vi "HFRR ADV v11.vi"() -> ()   [LabVIEW 2025] (continued)
          }
          frame True {
            (unwired) i16 6 ("width (-)")
            (unwired) "TESTED BY : "
            (unwired) "TESTED DATE :"
            (unwired) "SAMPLE ID : "
            (unwired) "SAMPLE DESIGN : "
            w4285 = "\r"
            w4302 = "\r"
            # "add image"
            n3133 = local read "Sample ID"() -> (w4275:string)
            n3134 = local read "Tested by"() -> (w4278:string)
            n3135 = local read "String 34"() -> (w4265:string)
            n3136 = local read "String 45"() -> (w4245:string)
            n3137 = local read "String 35"() -> (w4260:string)
            n3138 = local read "String 37"() -> (w4258:string)
            n3139 = local read "String 32"() -> (w4280:string)
            n3140 = local read "String 36"() -> (w4255:string)
            n3141 = local read "String 31"() -> (w4279:string)
            n3142 = local read "Test Date"() -> (w4276:string)
            n3143 = local read "String 33"() -> (w4281:string)
            n3144 = local read "String 38"() -> (w4251:string)
            n3145 = local read "String 39"() -> (w4248:string)
            n3146 = local write "Print"(FALSE ("Print FF")) -> ()
            n3147 = local read "S 39"() -> (w4263:string)
            n3148 = local read "S 38"() -> (w4270:string)
            n3149 = local read "Temperature before test 2"() -> (w4301:dbl)
            n3150 = local read "Temperature after test 2"() -> (w4291:dbl)
            n3151 = local read "Humidity before test 2"() -> (w4316:dbl)
            n3152 = local read "Humidity after test 2"() -> (w4300:dbl)
            n3153 = local read "MWSD 2"() -> (w4305:dbl)
            n3154 = local read "WS1.4 2"() -> (w4283:dbl)
            n3155 = Concatenate Strings("2)" ("string"), w4265) -> (w4266:string)
            n3156 = Concatenate Strings("3)" ("string"), w4263) -> (w4264:string)
            n3157 = Concatenate Strings("1)" ("string"), w4270) -> (w4269:string)
            n3158 = Concatenate Strings("4)" ("string"), w4260) -> (w4261:string)
            n3159 = Concatenate Strings("5)" ("string"), w4258) -> (w4257:string)
            n3160 = Concatenate Strings("6)" ("string"), w4255) -> (w4254:string)
            n3161 = Concatenate Strings("7)" ("string"), w4251) -> (w4252:string)
            n3162 = Concatenate Strings("8)" ("string"), w4248) -> (w4249:string)
            n3163 = local read "HCF 2"() -> (w4287:dbl)
            n3164 = local read "AVP 2"() -> (w4304:dbl)
            n3165 = local read "s.NO"() -> (w4246:string)
            n3166 = call <vilib>:"New Report.vi"("report type"=enum16{"Standard Report", "HTML"}."Standard Report") -> ("report out"=w4325:refnum<class "NI_report.lvclass">, "error out"=w4324:errorcluster)  [unwired: 13 in]
            n3167 = local read "TITTLE"() -> (w4277:string)
            n3168 = Concatenate Strings(w4302, w4245, w4246, w4302, w4280, w4275, w4302, w4279, w4276, w4302, w4281, w4278, w4302) -> (w4295:string)
            "test by" <- w4295
            n3169 = Number To Fractional String(number=w4301, width (-)=i16 6, precision (6)=i16 2) -> (F-format string=w4290:string)  [unwired: 1 in]
            n3170 = Number To Fractional String(number=w4300, width (-)=i16 6, precision (6)=i16 2) -> (F-format string=w4303:string)  [unwired: 1 in]
            n3171 = Number To Fractional String(number=w4316, width (-)=i16 6, precision (6)=i16 2) -> (F-format string=w4321:string)  [unwired: 1 in]
            n3172 = Number To Fractional String(number=w4305, width (-)=i16 6, precision (6)=i16 2) -> (F-format string=w4307:string)  [unwired: 1 in]
            n3173 = Number To Fractional String(number=w4291, width (-)=i16 6, precision (6)=i16 2) -> (F-format string=w4292:string)  [unwired: 1 in]
            n3174 = Number To Fractional String(number=w4304, width (-)=i16 6, precision (6)=i16 2) -> (F-format string=w4306:string)  [unwired: 1 in]
            n3175 = Number To Fractional String(number=w4287, width (-)=i16 6, precision (6)=i16 2) -> (F-format string=w4286:string)  [unwired: 1 in]
            n3176 = Number To Fractional String(number=w4283, precision (6)=i16 2) -> (F-format string=w4282:string)  [unwired: 2 in]
            n3177 = call-dynamic "Set Report Header Text.vi"("report in"=w4325, "center header text"=w4277, "error in (no error)"=w4324) -> ("report out"=w4296:refnum<class "NI_report.lvclass">, "error out"=w4297:errorcluster)  [unwired: 11 in]
            n3178 = Concatenate Strings(w4285, w4269, w4321, w4285, w4266, w4290, w4285, w4264, w4303, w4285, w4261, w4292, w4285, w4257, w4307, w4285, w4254, w4306, w4285, w4252, w4286, w4285, w4249, w4282) -> (w4273:string)
            "export 2" <- w4273
            n3179 = call-poly <vilib>:"Append Report Text.vi"("report in"=w4296, "text"=w4295, "error in (no error)"=w4297) -> ("report out"=w4299:refnum<class "NI_report.lvclass">, "error out"=w4298:errorcluster)  [unwired: 9 in, 2 out]
            n3180 = local read "test by"() -> (w4272:string)
            n3181 = local read "TITTLE"() -> (w4274:string)
            n3182 = call-poly <vilib>:"Append Report Text.vi"("report in"=w4299, "error in (no error)"=w4298) -> ("report out"=w4320:refnum<class "NI_report.lvclass">, "error out"=w4318:errorcluster)  [unwired: 10 in, 2 out]
            n3183 = Concatenate Strings(w4274, w4273, w4272) -> (→"output":string)
            n3184 = call-poly <vilib>:"Append Report Text.vi"("report in"=w4320, "text"=w4273, "error in (no error)"=w4318) -> ("report out"=w4319:refnum<class "NI_report.lvclass">, "error out"=w4317:errorcluster)  [unwired: 9 in, 2 out]
            n3185 = call-dynamic "Print Report.vi"("report in"=w4319, "printer name (default)"=w4327, "error in (no error)"=w4317) -> ("report out"=w4329:refnum<class "NI_report.lvclass">, "error out"=w4330:errorcluster)  [unwired: 11 in]
            n3186 = call-dynamic "Dispose Report.vi"("report in"=w4329, "error in (no error)"=w4330) -> ()  [unwired: 13 in, 1 out]
          }
        }
        n3187 = case shown="True" "Print 2" {
          frame False {
          }
          frame True {
            n3188 = flat-sequence {
              frame #0 {
                n3189 = local read "s.NO"() -> (→"s.NO 2":string)
                n3190 = Wait (ms)(milliseconds to wait=u32 20) -> ()  [unwired: 1 out]
                n3191 = local read "Sample ID  3"() -> (→"Sample ID  6":string)
                n3192 = local read "Sample ID  4"() -> (→"Sample ID  7":string)
                n3193 = local read "Sample ID"() -> (→"Sample ID  2":string)
                n3194 = local read "Tested by"() -> (→"Tested by 2":string)
                n3195 = local read "Test Date"() -> (→"Test Date 2":string)
                n3196 = local read "Humidity after test 3"() -> (→"Humidity after test 4":dbl)
                n3197 = local read "Ref A Test Date :"() -> (→"TITTLE 4":string)
                n3198 = local read "Temperature before test 3"() -> (w4152:dbl)
                n3199 = local read "Temperature before test 3"() -> (→"Temperature after test 5":dbl)
                n3200 = local read "Temperature after test 3"() -> (→"Temperature after test 4":dbl)
                n3201 = local read "Humidity before test 3"() -> (→"Humidity before test 4":dbl)
                n3202 = local write "Temperature before test 3"(w4152) -> ()
                n3203 = local read "image data"() -> (w4143:T14)
                n3204 = String To Path(string="C:\\LAB-IQ\\im\\Temp_resized.jpg") -> (path=w4144:path)
                "path 2" <- w4144
                n3205 = call <vilib>:"Write JPEG File.vi"("image data"=w4143, "path to JPEG file"=w4144) -> ()  [unwired: 8 in, 2 out]
                "Ref A Test Date :" <- "Ref A Test Date :"
                "Ref B Test Date :" <- "Ref B Test Date :"
                "Ref B Scar Value :" <- "Ref B Scar Value :"
                "Ref A Scar Value :" <- "Ref A Scar Value :"
              }
              frame #1 {
                (unwired) HTML_Report_Image_Alignment."MIDDLE" ("alignment (default)")
                w4180 = u16 0 items=["portrait", "landscape"] ("orientation (portrait)")
                (unwired) HTML_Report_Image_Alignment."ABSMIDDLE" ("alignment (default)")
                (unwired) "TESTED BY : "
                (unwired) "TESTED DATE :"
                (unwired) "SAMPLE ID : "
                (unwired) "SAMPLE DESIGN : "
                w4213 = "\r"
                # "add image"
                n3206 = Wait (ms)(milliseconds to wait=u32 20) -> ()  [unwired: 1 out]
                n3207 = local read "Sample ID  2"() -> (w4206:string)
                n3208 = local read "Wear Scar X"() -> (w4178:dbl)
                "Length ( microns ) 2" <- w4178
                n3209 = local read "Wear Scar Y"() -> (w4177:dbl)
                "Wear Scar Y ( microns ) :" <- w4177
                n3210 = local read "Test Date 2"() -> (w4207:string)
                n3211 = local read "Tested by 2"() -> (w4208:string)
                n3212 = local read "String 46"() -> (w4204:string)
                n3213 = local read "String 48"() -> (w4210:string)
                n3214 = local read "String 47"() -> (w4209:string)
                n3215 = local read "String 49"() -> (w4211:string)
                n3216 = local read "String 10"() -> (w4164:string)
                n3217 = local read "s.NO 2"() -> (w4205:string)
                n3218 = Add(x=w4178, y=w4177) -> (x+y=w4176:dbl)
                n3219 = call <vilib>:"New Report.vi"("report type"=enum16{"Standard Report", "HTML"}."HTML") -> ("report out"=w4184:refnum<class "NI_report.lvclass">, "error out"=w4182:errorcluster)  [unwired: 13 in]
                n3220 = Concatenate Strings(w4213, w4204, w4205, w4213, w4210, w4206, w4213, w4209, w4207, w4213, w4211, w4208, w4213) -> (→"test by 2":string)
                n3221 = Concatenate Strings("C:\\LAB-IQ\\Data\\" ("string"), w4164, ".jpg" ("string")) -> ()  [unwired: 1 out]
                n3222 = Divide(x=w4176, y=2.0) -> (x/y=→"Mean Wear ( microns) :":dbl)
                n3223 = call-dynamic "Set Report Orientation.vi"("report in"=w4184, "orientation (portrait)"=w4180, "error in (no error)"=w4182) -> ("report out"=w4183:refnum<class "NI_report.lvclass">, "error out"=w4181:errorcluster)  [unwired: 11 in]
                n3224 = for {
                  N: 5 -> [_]
                  tunnel: w4183 -> [w4234]
                  tunnel: [w4233] -> w4162
                  tunnel: w4181 -> [w4232]
                  tunnel: [w4231] -> w4161
                  n3225 = call-dynamic "Set Report Tab Width.vi"("report in"=w4234, "error in (no error)"=w4232) -> ("report out"=w4233:refnum<class "NI_report.lvclass">, "error out"=w4231:errorcluster)  [unwired: 12 in]
                }
                n3226 = local read "TITTLE"() -> (w4179:string)
                n3227 = call-dynamic "Set Report Header Text.vi"("report in"=w4162, "center header text"=w4179, "error in (no error)"=w4161) -> ("report out"=w4200:refnum<class "NI_report.lvclass">, "error out"=w4199:errorcluster)  [unwired: 11 in]
                n3228 = for {
                  N: 1 -> [_]
                  tunnel: [w4238] -> w4186
                  tunnel: [w4237] -> w4185
                  tunnel: w4200 -> [w4236]
                  tunnel: w4199 -> [w4235]
                  n3229 = call-dynamic "New Report Line.vi"("report in"=w4236, "error in (no error)"=w4235) -> ("report out"=w4238:refnum<class "NI_report.lvclass">, "error out"=w4237:errorcluster)  [unwired: 12 in]
                }
                n3230 = for {
                  N: 2 -> [_]
                  tunnel: [w4230] -> w4192
                  tunnel: [w4229] -> w4191
                  tunnel: w4186 -> [w4228]
                  tunnel: w4185 -> [w4227]
                  n3231 = call-dynamic "New Report Line.vi"("report in"=w4228, "error in (no error)"=w4227) -> ("report out"=w4230:refnum<class "NI_report.lvclass">, "error out"=w4229:errorcluster)  [unwired: 12 in]
                }
                n3232 = for {
                  N: 25 -> [_]
                  tunnel: w4192 -> [w4226]
                  tunnel: w4191 -> [w4224]
                  tunnel: [w4225] -> w4195
                  tunnel: [w4223] -> w4194
                  n3233 = call-dynamic "Set Report Tab Width.vi"("report in"=w4226, "error in (no error)"=w4224) -> ("report out"=w4225:refnum<class "NI_report.lvclass">, "error out"=w4223:errorcluster)  [unwired: 12 in]
                }
                n3234 = control-ref of="Tab Control 9"() -> (w4190:refnum<vi>)
                n3235 = call-dynamic "Append Control Image to Report.vi"("report in"=w4195, "alignment (default)"=HTML_Report_Image_Alignment."ABSMIDDLE", "ctrl reference"=w4190, "error in (no error)"=w4194) -> ("report out"=w4189:refnum<class "NI_report.lvclass">, "error out"=w4188:errorcluster)  [unwired: 8 in, 2 out]
                n3236 = for {
                  N: 3 -> [_]
                  tunnel: [w4222] -> w4173
                  tunnel: [w4221] -> w4172
                  tunnel: w4189 -> [w4220]
                  tunnel: w4188 -> [w4219]
                  n3237 = call-dynamic "New Report Line.vi"("report in"=w4220, "error in (no error)"=w4219) -> ("report out"=w4222:refnum<class "NI_report.lvclass">, "error out"=w4221:errorcluster)  [unwired: 12 in]
                }
                n3238 = for {
                  N: 100 -> [_]
                  tunnel: w4173 -> [w4218]
                  tunnel: w4172 -> [w4216]
                  tunnel: [w4217] -> w4169
                  tunnel: [w4215] -> w4167
                  n3239 = call-dynamic "Set Report Tab Width.vi"("report in"=w4218, "error in (no error)"=w4216) -> ("report out"=w4217:refnum<class "NI_report.lvclass">, "error out"=w4215:errorcluster)  [unwired: 12 in]
                }
                n3240 = String To Path(string="C:\\LAB-IQ\\im\\Temp_resized.jpg") -> (path=w4159:path)
                n3241 = call-poly <vilib>:"Append Image to Report.vi"("report in"=w4169, "path or URL of image"=w4159, "error in (no error)"=w4167) -> ("report out"=w4168:refnum<class "NI_report.lvclass">, "error out"=w4166:errorcluster)  [unwired: 9 in, 2 out]
                n3242 = call-poly <vilib>:"Open HTML Report in Browser.vi"("report in"=w4168, "error in (no error)"=w4166) -> ("report out"=w4203:refnum<class "NI_report.lvclass">, "error out"=w4202:errorcluster)  [unwired: 11 in, 1 out]
                n3243 = call-dynamic "Dispose Report.vi"("report in"=w4203, "error in (no error)"=w4202) -> ()  [unwired: 13 in, 1 out]
              }
              frame #2 {
              }
              frame #3 {
                n3244 = disable-structure shown="Disabled" {
                  frame Disabled {
                    n3245 = local read "String 10"() -> (w4243:string)
                    n3246 = Concatenate Strings("C:\\LAB-IQ-NXT\\Data\\" ("string"), w4243, ".jpg" ("string")) -> (w4241:string)
                    n3247 = String To Path(string=w4241) -> (path=w4240:path)
                    n3248 = Delete(path (use dialog)=w4240) -> ()  [unwired: 4 in, 3 out]
                  }
                  frame Enabled {
                  }
                }
                n3249 = local write "Print 2"(FALSE ("Print")) -> ()
              }
            }
          }
        }
      }
    }
    n3250 = property on="SetTemp" class="DigNum (strict)"("Disabled"=w2127) -> ()  [unwired: 2 in, 2 out]
    n3251 = Multiply(x=w2116, y=w2118) -> (x*y=w2117:dbl)
    n3252 = local read "MWSD"() -> (w2115:dbl)
    n3253 = Add(x=w2117, y=w2115) -> (x+y=→"WS1.4":dbl)
    n3254 = Wait (ms)(milliseconds to wait=u32 50) -> ()  [unwired: 1 out]
    n3255 = Wait (ms)(milliseconds to wait=u32 50) -> ()  [unwired: 1 out]
    n3256 = local read "Quit"() -> (w2114:bool)
  }
  n3257 = VISA Close(VISA resource name=w53, error in (no error)=w52) -> (error out=w50:errorcluster)
  n3258 = VISA Close(VISA resource name=w34, error in (no error)=w33) -> ()  [unwired: 1 out]
  n3259 = call <vilib>:"Clear Errors.vi"("error in (no error)"=w50) -> ()  [unwired: 5 in, 2 out]
  n3260 = Or(x=w40, y=w39) -> (x .or. y?=w41:bool)
  n3261 = while {
    tunnel: [w4391] -> w46
    shift-right: [w4429] -> _
    shift-left: "" -> [w4417]
    tunnel: [w4405] -> _
    i -> [w4405]
    stop <- w4391 stop-if-true
    w4431 = ";" ("string")
    n3262 = local read "start en"() -> (w4450:bool)
    n3263 = And(x="st enable", y=w4450) -> (x .and. y?=w4451:bool)
    n3264 = local read "Elapsed time"() -> (w4413:dbl)
    n3265 = local read "ACQUIRE 3"() -> (w4394:bool)
    n3266 = case shown="True" w4451 {
      tunnel: "st enable" -> [w4515 w4516]
      tunnel: [w4515 w4516] -> w4395
      frame False {
      }
      frame True {
        n3267 = local write "start en"(FALSE ("start en")) -> ()
      }
    }
    n3268 = Wait (ms)(milliseconds to wait=u32 80) -> ()  [unwired: 1 out]
    n3269 = local read "Stroke"() -> (w4404:dbl)
    n3270 = Greater?(x=w4413, y=0.1) -> (0:w4411:bool)
    n3271 = Or(x=w4395, y=w4394) -> (x .or. y?=w4396:bool)
    n3272 = case shown="True" "ACQUIRE 2" {
      frame False {
      }
      frame True {
        n3273 = call "Elapsed Time13"() -> ("Time has Elapsed"=w4458:bool)  [unwired: 12 in, 7 out]
        n3274 = case shown="True" w4458 {
          frame False {
          }
          frame True {
            n3275 = local write "ACQUIRE 2"(FALSE ("ACQUIRE 2")) -> ()
            n3276 = local write "ACQUIRE 3"(FALSE ("ACQUIRE 2")) -> ()
          }
        }
        n3277 = local write "ACQUIRE 3"(TRUE ("ACQUIRE 2")) -> ()
      }
    }
    n3278 = case shown="True" w4396 {
      tunnel: w4404 -> [_ w4538]
      tunnel: [w4518 _] -> w4448
      tunnel: w4411 -> [_ _]
      tunnel: w4394 -> [_ w4525]
      frame False {
        w4518 = TRUE ("PID Rst")
        n3279 = local read "stop cmd"() -> (w4519:bool)
        n3280 = case shown="True" w4519 {
          frame False {
          }
          frame True {
            n3281 = local write "stop cmd"(FALSE ("stop cmd")) -> ()
          }
        }
        n3282 = local write "PID Rst"(TRUE ("PID Rst")) -> ()
        "start en" <- w4518
      }
      frame True {
        w4545 = cluster{"output high":dbl, "output low":dbl} {"output high"=600.0, "output low"=-600.0} ("output range")
        n3283 = local read "STROKE GAIN :"() -> (w4530:dbl)
        n3284 = call "Elapsed Time6"("Reset"="PID Rst", "Auto Reset"=FALSE) -> ("Time has Elapsed"=w4539:bool)  [unwired: 10 in, 7 out]
        n3285 = Multiply(x="Set Strk", y=w4530) -> (x*y=w4523:dbl)
        n3286 = case shown="False" w4539 {
          tunnel: [w4550 w4551] -> w4542
          tunnel: "Set Strk" -> [w4550 _]
          tunnel: w4538 -> [_ w4551]
          frame False {
          }
          frame True {
          }
        }
        n3287 = Multiply(x=w4523, y=1.0) -> (x*y=w4522:dbl)
        n3288 = Select(t=T9 {"Proportional Gain (Kc)"=0.0, "Integral Time (Ti, min)"=0.02, "Derivative Time (Td, min)"=0.0} ("Stroke PID Gains"), s=w4525, f="Stroke PID Gains") -> (s? t:f=w4526:T9)
        n3289 = Not(x=w4539) -> (.not. x?=w4537:bool)
        n3290 = call-poly <vilib>:"PID.vi"("reinitialize? (F)"=w4537, "output range"=w4545, "PID gains"=w4526, "process variable"=w4542, "setpoint"="Set Strk") -> ("output"=w4536:dbl)  [unwired: 5 in, 1 out]
        "Stroke PID OUT" <- w4536
        n3291 = Select(t=w4536, s=w4539, f=0.0) -> (s? t:f=w4540:dbl)
        n3292 = flat-sequence {
          tunnel: w4540 -> [_]
          frame #0 {
            n3293 = local write "PID Rst"(FALSE ("PID Rst")) -> ()
          }
        }
        n3294 = Add(x=w4522, y=w4540) -> (x+y=w4535:dbl)
        n3295 = Unbundle(w4545) -> ("output high"=w4544:dbl, "output low"=w4543:dbl)
        n3296 = To Word Integer(number=w4535) -> (16bit integer=w4532:i16)
        n3297 = property on="Stroke PID OUT" class="Slide (strict)"("Scale.Range:Minimum"=w4543, "Scale.Range:Maximum"=w4544) -> ()  [unwired: 2 in, 2 out]
        n3298 = In Range and Coerce(upper limit=4095.0 ("f"), x=w4532, lower limit=100.0 ("f")) -> (coerced(x)=w4529:dbl)  [unwired: 1 out]
        "PID Out" <- w4529
        n3299 = Number To Decimal String(number=w4529) -> (decimal integer string=→"st gain":string)  [unwired: 1 in]
        "stop cmd" <- TRUE ("Auto Reset")
      }
    }
    n3300 = flat-sequence {
      frame #0 {
        n3301 = local read "CH-POWER +"() -> (w4462:u16)
        n3302 = local read "CH-POWER -"() -> (w4463:u16)
        n3303 = case shown="1" w4463 {
          tunnel: "PWR" -> [w4464 w4465 w4466 w4467 w4468 w4469 w4470 w4471]
          frame 0, Default {
            n3304 = local write "Do 0"(w4464) -> ()
          }
          frame 1 {
            n3305 = local write "Do 1"(w4465) -> ()
          }
          frame 2 {
            n3306 = local write "Do 2"(w4466) -> ()
          }
          frame 3 {
            n3307 = local write "Do 3"(w4467) -> ()
          }
          frame 4 {
            n3308 = local write "Do 4"(w4468) -> ()
          }
          frame 5 {
            n3309 = local write "Do 5"(w4469) -> ()
          }
          frame 6 {
            n3310 = local write "Do 6"(w4470) -> ()
          }
          frame 7 {
            n3311 = local write "Do 7"(w4471) -> ()
          }
        }
        n3312 = case shown="1" w4462 {
          tunnel: "PWR" -> [w4472 w4473 w4474 w4475 w4476 w4477 w4478 w4479]
          frame 0, Default {
            n3313 = local write "Do 0"(w4472) -> ()
          }
          frame 1 {
            n3314 = local write "Do 1"(w4473) -> ()
          }
          frame 2 {
            n3315 = local write "Do 2"(w4474) -> ()
          }
          frame 3 {
            n3316 = local write "Do 3"(w4475) -> ()
          }
          frame 4 {
            n3317 = local write "Do 4"(w4476) -> ()
          }
          frame 5 {
            n3318 = local write "Do 5"(w4477) -> ()
          }
          frame 6 {
            n3319 = local write "Do 6"(w4478) -> ()
          }
          frame 7 {
            n3320 = local write "Do 7"(w4479) -> ()
          }
        }
      }
    }
    n3321 = local read "RUN"() -> (w4402:bool)
    n3322 = Or(x=w4402, y="ACQUIRE 3") -> (x .or. y?=w4401:bool)
    n3323 = local read "Set Hz"() -> (w4419:dbl)
    n3324 = Select(t=w4419, s=w4401, f=0.0) -> (s? t:f=w4418:dbl)
    n3325 = local read "st gain"() -> (w4422:string)
    n3326 = local read "DO"() -> (w4423:string)
    n3327 = case shown="True" "Boolean 10" {
      frame False {
      }
      frame True {
        n3328 = local write "Tab Control 8"(enum32{"setup", "calibrate"}."calibrate" ("Tab Control 8")) -> ()
        n3329 = local write "Boolean 10"(FALSE ("Boolean 10")) -> ()
      }
    }
    n3330 = Number To Decimal String(number=w4418) -> (decimal integer string=w4421:string)  [unwired: 1 in]
    n3331 = case shown="True" "Boolean 11" {
      frame False {
      }
      frame True {
        n3332 = local write "Tab Control 8"(enum32{"setup", "calibrate"}."setup" ("Tab Control 8")) -> ()
        n3333 = local write "Boolean 11"(FALSE ("Boolean 11")) -> ()
      }
    }
    n3334 = String Length(string=w4422) -> (length=w4437:i32)
    n3335 = String Length(string=w4423) -> (length=w4425:i32)
    n3336 = String Length(string=w4421) -> (length=w4438:i32)
    n3337 = Subtract(x=4.0, y=w4437) -> (x-y=w4434:dbl)
    n3338 = Subtract(x=3.0, y=w4425) -> (x-y=w4428:dbl)
    n3339 = flat-sequence {
      tunnel: w4448 -> [_]
      frame #0 {
        n3340 = Build Array("Do 0", "Do 1", "Do 2", "Do 3", "Do 4", "Do 5", "Do 6", "Do 7") -> (w4506:bool[])
        n3341 = Boolean Array To Number(Boolean array=w4506) -> (number=w4504:u32)
        n3342 = Add(x=w4504, y=u32 0) -> (x+y=w4502:u32)
        n3343 = Number To Decimal String(number=w4502) -> (decimal integer string=→"DO":string)  [unwired: 1 in]
      }
    }
    n3344 = Subtract(x=3.0, y=w4438) -> (x-y=w4439:dbl)
    n3345 = Replace Substring(3:w4434, 4:w4422, 5:"0000" ("string")) -> (1:w4432:string)  [unwired: 1 in, 1 out]
    n3346 = Replace Substring(3:w4428, 4:w4423, 5:"000" ("string")) -> (1:w4424:string)  [unwired: 1 in, 1 out]
    n3347 = Replace Substring(3:w4439, 4:w4421, 5:"000" ("string")) -> (1:w4433:string)  [unwired: 1 in, 1 out]
    n3348 = Concatenate Strings("*" ("string"), w4433, w4431, w4432, w4431, w4424, "$" ("string")) -> (w4429:string)
    "Stroke_send_Val" <- w4429
    n3349 = local read "RUN"() -> (w4399:bool)
    n3350 = local read "ACQUIRE 3"() -> (w4398:bool)
    n3351 = local read "send"() -> (w4415:bool)
    n3352 = Not Equal?(x=w4417, y=w4429) -> (x != y?=w4430:bool)
    n3353 = Or(x=w4399, y=w4398) -> (x .or. y?=w4397:bool)
    n3354 = And(x=w4415, y=w4397) -> (x .and. y?=w4414:bool)
    n3355 = Or(x=w4430, y=w4414) -> (x .or. y?=w4408:bool)
    n3356 = case shown="False" w4397 {
      frame False {
        "send" <- TRUE ("send")
      }
      frame True {
      }
    }
    n3357 = call "Elapsed Time4"("Time Target (s)"=0.5) -> ("Time has Elapsed"=w4406:bool)  [unwired: 11 in, 7 out]
    n3358 = local read "Din"() -> (w4447:u8[])
    n3359 = Or(x=w4406, y=w4408) -> (x .or. y?=w4407:bool)
    n3360 = local read "Quit"() -> (w4391:bool)
    n3361 = Index Array(array=w4447, index=0) -> (element=w4445:u8)
    n3362 = case shown="True" w4407 {
      tunnel: w4429 -> [_ w4483]
      frame False {
      }
      frame True {
        n3363 = local read "Due Com"() -> (w4484:string[])
        n3364 = Build Array (concatenate)(w4484, w4483) -> (→"Due Com":string[])
        n3365 = local write "send"(FALSE ("send")) -> ()
      }
    }
    n3366 = Number To Boolean Array(number=w4445) -> (Boolean array=w4444:bool[])
    n3367 = Array Size(array=w4444) -> (size(s)=w4443:i32)
    n3368 = Greater Than 0?(x=w4443) -> (x > 0?=w4442:bool)
    n3369 = case shown="True" w4442 {
      tunnel: w4444 -> [_ w4498]
      frame False {
      }
      frame True {
        n3370 = Index Array(array=w4498, index #1=0 ("index"), index #2=1 ("index"), index #3=2 ("index"), index #4=3 ("index"), index #5=4 ("index"), index #6=5 ("index"), index #7=6 ("index"), index #8=7 ("index")) -> (element #1=→"DI 0":bool, element #2=→"DI 1":bool, element #3=→"DI 2":bool, element #4=→"DI 3":bool, element #5=→"DI 4":bool, element #6=→"DI 5":bool, element #7=→"DI 6":bool, element #8=→"DI 7":bool)
      }
    }
  }
  n3371 = Or(x=w36, y=w41) -> (x .or. y?=w48:bool)
  n3372 = control-ref of="new picture"() -> ()  [unwired: 1 out]
  n3373 = Or(x=w55, y=w48) -> (x .or. y?=w45:bool)
  n3374 = Or(x=w45, y=w46) -> (x .or. y?=w37:bool)
  n3375 = while {
    tunnel: [w4553] -> w59
    tunnel: [w4554] -> _
    i -> [w4554]
    stop <- w4553 stop-if-true
    n3376 = local read "PID-out"() -> (w4555:dbl)
    "Horizontal Slider Control" <- w4555
    n3377 = Greater Or Equal?(x=w4555, y=2.0) -> (x >= y?=w4556:bool)
    n3378 = flat-sequence {
      tunnel: w4556 -> [w4564]
      tunnel: w4555 -> [w4567]
      tunnel: [w4565] -> w4562
      tunnel: [w4563] -> w4561
      tunnel: [w4583] -> w4560
      tunnel: w4562 -> [w4583]
      tunnel: w4561 -> [w4580]
      tunnel: [w4580] -> w4559
      tunnel: w4560 -> [w4585]
      tunnel: [w4584] -> w4558
      tunnel: w4559 -> [w4584]
      tunnel: w4558 -> [w4599]
      frame #0 {
        n3379 = case shown="True" w4564 {
          selector: w4564 -> [w4569 _]
          frame False {
            n3380 = local write "HEATER"(w4569) -> ()
          }
          frame True {
            w4571 = TRUE ("data")
            n3381 = local read "CH-HEATER"() -> (w4570:u16)
            n3382 = case shown="2" w4570 {
              tunnel: w4571 -> [w4572 w4573 w4574 w4575 w4576 w4577 w4578 w4579]
              frame 0, Default {
                n3383 = local write "Do 0"(w4572) -> ()
              }
              frame 1 {
                n3384 = local write "Do 1"(w4573) -> ()
              }
              frame 2 {
                n3385 = local write "Do 2"(w4574) -> ()
              }
              frame 3 {
                n3386 = local write "Do 3"(w4575) -> ()
              }
              frame 4 {
                n3387 = local write "Do 4"(w4576) -> ()
              }
              frame 5 {
                n3388 = local write "Do 5"(w4577) -> ()
              }
              frame 6 {
                n3389 = local write "Do 6"(w4578) -> ()
              }
              frame 7 {
                n3390 = local write "Do 7"(w4579) -> ()
              }
            }
            "HEATER" <- w4571
          }
        }
        n3391 = Select(t=w4567, s=w4564, f=0.0) -> (s? t:f=w4563:dbl)
        n3392 = Greater Or Equal?(x=w4567, y=97.0) -> (x >= y?=w4565:bool)
      }
      frame #1 {
        n3393 = Multiply(x=w4580, y=5.0) -> (x*y=w4582:dbl)
        n3394 = Wait (ms)(milliseconds to wait=w4582) -> ()  [unwired: 1 out]
      }
      frame #2 {
        n3395 = case shown="False" w4585 {
          frame False {
            w4586 = FALSE ("data")
            n3396 = local read "CH-HEATER"() -> (w4587:u16)
            n3397 = case shown="4" w4587 {
              tunnel: w4586 -> [w4588 w4589 w4590 w4591 w4592 w4593 w4594 w4595]
              frame 0, Default {
                n3398 = local write "Do 0"(w4588) -> ()
              }
              frame 1 {
                n3399 = local write "Do 1"(w4589) -> ()
              }
              frame 2 {
                n3400 = local write "Do 2"(w4590) -> ()
              }
              frame 3 {
                n3401 = local write "Do 3"(w4591) -> ()
              }
              frame 4 {
                n3402 = local write "Do 4"(w4592) -> ()
              }
              frame 5 {
                n3403 = local write "Do 5"(w4593) -> ()
              }
              frame 6 {
                n3404 = local write "Do 6"(w4594) -> ()
              }
              frame 7 {
                n3405 = local write "Do 7"(w4595) -> ()
              }
            }
            n3406 = local write "HEATER"(w4586) -> ()
          }
          frame True {
          }
        }
      }
      frame #3 {
        n3407 = Subtract(x=100, y=w4599) -> (x-y=w4598:dbl)
        n3408 = Multiply(x=w4598, y=5.0) -> (x*y=w4596:dbl)
        n3409 = Wait (ms)(milliseconds to wait=w4596) -> ()  [unwired: 1 out]
      }
    }
    n3410 = local read "Quit"() -> (w4553:bool)
  }
  n3411 = Or(x=w59, y=w37) -> (x .or. y?=w58:bool)
  n3412 = while {
    tunnel: [w4601] -> w54
    i -> [w4608]
    stop <- w4601 stop-if-true
    n3413 = local read "Quit"() -> (w4601:bool)
    n3414 = Equal To 0?(x=w4608) -> (x = 0?=w4606:bool)
    n3415 = call "Elapsed Time3"("Time Target (s)"=45.0, "Auto Reset"=TRUE) -> ("Time has Elapsed"=w4605:bool)  [unwired: 10 in, 7 out]
    n3416 = Wait (ms)(milliseconds to wait=u32 50) -> ()  [unwired: 1 out]
    n3417 = Or(x=w4605, y=w4606) -> (x .or. y?=w4607:bool)
    n3418 = case shown="True" w4607 {
      frame False {
      }
      frame True {
        n3419 = call <vilib>:"System Exec.vi"("run minimized? (F)"=TRUE, "error in (no error)"="error in (no error)", "command line"="powercfg.exe -change -monitor-timeout-ac 0") -> ("error out"=w4619:errorcluster)  [unwired: 5 in, 3 out]
        n3420 = call <vilib>:"System Exec.vi"("run minimized? (F)"=TRUE, "error in (no error)"=w4619, "command line"="powercfg.exe -change -disk-timeout-ac 0") -> ("error out"=w4618:errorcluster)  [unwired: 5 in, 3 out]
        n3421 = call <vilib>:"System Exec.vi"("run minimized? (F)"=TRUE, "error in (no error)"=w4618, "command line"="powercfg.exe -change -standby-timeout-ac 0") -> ("error out"=w4617:errorcluster)  [unwired: 5 in, 3 out]
        n3422 = call <vilib>:"System Exec.vi"("run minimized? (F)"=TRUE, "error in (no error)"=w4617, "command line"="powercfg.exe -change -hibernate-timeout-ac 0") -> ("error out"=w4616:errorcluster)  [unwired: 5 in, 3 out]
        n3423 = call <vilib>:"Simple Error Handler.vi"("error in (no error)"=w4616) -> ("error out"=w4622:errorcluster)  [unwired: 4 in, 4 out]
        n3424 = call <vilib>:"Clear Errors.vi"("error in (no error)"=w4622) -> ("error out"=→"error out":errorcluster)  [unwired: 5 in, 1 out]
      }
    }
  }
  n3425 = Compound Arithmetic op=OR(w57, w58, w54) -> (w56:bool)
  n3426 = flat-sequence {
    tunnel: w56 -> [_]
    tunnel: [w4624] -> w14
    tunnel: w14 -> [_]
    frame #0 {
      n3427 = call "CLOSE CONNECTION.vi"() -> ("error out"=w4624:errorcluster)  [unwired: 11 in]
    }
    frame #1 {
      n3428 = Quit LabVIEW(quit? (T)=TRUE) -> ()
      n3429 = local write "Quit"(FALSE ("EXIT")) -> ()
    }
  }
  n3430 = property on="Heater Button" class="Bool (strict)"("Visible"=TRUE) -> ()  [unwired: 2 in, 2 out]
  n3431 = disable-structure shown="Disabled" {
    disable-tunnel: _ -> [w4630 _]
    disable-tunnel: _ -> [w4627 _]
    disable-tunnel: _ -> [w4628 _]
    frame Disabled {
      n3432 = disable-structure shown="Disabled" {
        disable-tunnel: [w4637 _] -> w4629
        frame Disabled {
          n3433 = while {
            shift-right: [w4679] -> w4635
            shift-left: errorcluster {"status"=TRUE, "code"=0, "source"="Init"} ("error out") -> [w4644]
            shift-right: [w4678] -> w4634
            shift-left: _ -> [w4645]
            shift-right: [w4677] -> _
            shift-left: "" -> [w4676]
            tunnel: [w4638] -> w4637
            shift-right: ["Set Rh"] -> _
            shift-left: 0.0 ("Set Rh") -> [w4670]
            tunnel: [w4647] -> _
            i -> [w4647]
            stop <- w4638 stop-if-true
            n3434 = flat-sequence {
              tunnel: w4644 -> [w4682]
              tunnel: [w4682] -> w4643
              frame #0 {
                n3435 = Wait (ms)(milliseconds to wait=u32 200) -> ()  [unwired: 1 out]
              }
            }
            n3436 = local read "Com Port 3"() -> (w4646:refnum<visa-resource-name>)
            n3437 = local read "Humidity Str Rec"() -> (w4648:string)
            n3438 = Not Equal?(x="Set Rh", y=w4670) -> (x != y?=w4675:bool)
            n3439 = Number To Decimal String(number="Set Rh") -> (decimal integer string=w4673:string)  [unwired: 1 in]
            n3440 = Not Equal?(x=w4646, y=w4645) -> (x != y?=w4641:bool)
            n3441 = Concatenate Strings("#setPoint00" ("string"), w4673) -> (w4674:string)
            n3442 = case shown="False" w4675 {
              tunnel: w4674 -> [_ w4694]
              frame False {
                n3443 = local read "Humidity"() -> (w4691:bool)
                n3444 = case shown="True" w4691 {
                  frame False {
                    n3445 = local write "Humidity Str Send"("stop" ("Humidity Str Send")) -> ()
                  }
                  frame True {
                    n3446 = local write "Humidity Str Send"("start" ("Humidity Str Send")) -> ()
                  }
                }
              }
              frame True {
                n3447 = local write "Humidity Str Send"(w4694) -> ()
              }
            }
            n3448 = Or(x=w4641, y="Re-Initialise") -> (x .or. y?=w4640:bool)
            n3449 = String Subset(string=w4648, offset (0)=7) -> (substring=w4663:string)  [unwired: 1 in]
            n3450 = Match Pattern(string=w4648, regular expression="?") -> (offset past match=w4666:i32)  [unwired: 1 in, 3 out]
            n3451 = Match Pattern(string=w4648, regular expression="v") -> (offset past match=w4669:i32)  [unwired: 1 in, 3 out]
            n3452 = case shown="True" w4640 {
              tunnel: w4643 -> [w4680 _]
              tunnel: [w4680 errorcluster {"status"=TRUE, "code"=0, "source"="Init"} ("error out")] -> w4642
              frame False {
              }
              frame True {
              }
            }
            n3453 = Equal?(x=w4666, y=-1) -> (x = y?=w4650:bool)
            n3454 = Match Pattern(string=w4663, regular expression="g") -> (after substring=w4664:string, offset past match=w4655:i32)  [unwired: 1 in, 2 out]
            n3455 = Match Pattern(string=w4663, regular expression="y") -> (after substring=w4662:string, offset past match=w4656:i32)  [unwired: 1 in, 2 out]
            n3456 = Greater?(x=w4656, y=w4655) -> (0:w4661:bool)
            n3457 = Greater Or Equal To 0?(x=w4656) -> (x >= 0?=w4653:bool)
            n3458 = Greater Or Equal To 0?(x=w4655) -> (x >= 0?=w4654:bool)
            n3459 = Or(x=w4653, y=w4654) -> (x .or. y?=w4652:bool)
            n3460 = Greater Or Equal To 0?(x=w4669) -> (x >= 0?=w4651:bool)
            n3461 = Select(t=w4662, s=w4661, f=w4664) -> (s? t:f=w4657:string)
            n3462 = case shown="Error" w4642 {
              selector: w4642 -> [w4707 w4753]
              tunnel: [w4705 w4746] -> w4679
              tunnel: w4645 -> [w4708 w4752]
              tunnel: [w4706 w4755] -> w4678
              tunnel: w4676 -> [w4695 w4754]
              tunnel: [w4702 w4754] -> w4677
              frame No Error {
                n3463 = call "Elapsed Time7"() -> ("Time has Elapsed"=w4701:bool)  [unwired: 12 in, 7 out]
                n3464 = Not Equal?(x="Humidity Str Send", y=w4695) -> (x != y?=w4697:bool)
                n3465 = Or(x=w4697, y=w4701) -> (x .or. y?=w4700:bool)
                n3466 = Select(t="Humidity Str Send", s=w4697, f="vals" ("regular expression")) -> (s? t:f=w4696:string)
                n3467 = Or(x=w4700, y="Send") -> (x .or. y?=w4704:bool)
                n3468 = case shown="True" w4704 {
                  tunnel: [w4711 w4716] -> w4705
                  tunnel: w4708 -> [w4710 w4724]
                  tunnel: w4707 -> [w4711 w4723]
                  tunnel: [w4710 w4717] -> w4706
                  tunnel: w4696 -> [_ w4722]
                  tunnel: [w4709 w4713] -> w4702
                  tunnel: "Humidity Str Send" -> [_ w4714]
                  tunnel: w4697 -> [_ w4715]
                  tunnel: w4695 -> [w4709 w4712]
                  frame False {
                  }
                  frame True {
                    n3469 = flat-sequence {
                      tunnel: w4724 -> [w4732]
                      tunnel: w4723 -> [w4731]
                      tunnel: w4722 -> [w4728]
                      tunnel: [w4730] -> w4721
                      tunnel: [w4729] -> w4720
                      tunnel: w4721 -> [w4735]
                      tunnel: w4720 -> [w4734]
                      tunnel: [w4735] -> w4719
                      tunnel: [w4734] -> w4718
                      tunnel: w4719 -> [w4742]
                      tunnel: w4718 -> [w4741]
                      tunnel: [w4740] -> w4717
                      tunnel: [w4739] -> w4716
                      frame #0 {
                        n3470 = local write "Ser Led"(TRUE ("Boolean 4")) -> ()
                        n3471 = Concatenate Strings(w4728, "\r") -> (w4727:string)
                        n3472 = VISA Write(VISA resource name=w4732, write buffer=w4727, error in (no error)=w4731) -> (VISA resource name out=w4730:refnum<visa-resource-name>, error out=w4729:errorcluster)  [unwired: 1 out]
                      }
                      frame #1 {
                        n3473 = Wait (ms)(milliseconds to wait="wait") -> ()  [unwired: 1 out]
                      }
                      frame #2 {
                        w4737 = FALSE ("Send")
                        n3474 = property class="Instr"(reference=w4742, error in=w4741) -> (reference out=w4743:refnum<visa-resource-name>, error out=w4744:errorcluster, "Serial Settings:Number of Bytes at Serial Port"=w4736:u32)
                        "Humidity 2" <- w4736
                        n3475 = local write "Send"(w4737) -> ()
                        n3476 = local write "Ser Led"(w4737) -> ()
                        n3477 = VISA Read(VISA resource name=w4743, byte count=w4736, error in (no error)=w4744) -> (VISA resource name out=w4740:refnum<visa-resource-name>, read buffer=→"Humidity Str Rec":string, error out=w4739:errorcluster)  [unwired: 1 out]
                      }
                    }
                    n3478 = Select(t=w4714, s=w4715, f=w4712) -> (s? t:f=w4713:string)
                  }
                }
              }
              frame Error {
                w4760 = u16 0 items=["None"=0, "XON/XOFF"=1, "RTS/CTS"=2, "DTR/DSR"=4] ("flow control")
                w4756 = u16 0 items=["None", "Odd", "Even", "Mark", "Space"] ("parity")
                w4759 = u16 10 items=["1.0"=10, "1.5"=15, "2.0"=20] ("stop bits")
                n3479 = VISA Close(VISA resource name=w4752, error in (no error)=w4753) -> (error out=w4751:errorcluster)
                n3480 = local write "humid"("" ("humid")) -> ()
                n3481 = local write "Humidity Str Rec"("" ("Humidity Str Rec")) -> ()
                n3482 = call <vilib>:"Clear Errors.vi"("error in (no error)"=w4751) -> ("error out"=w4750:errorcluster)  [unwired: 5 in, 1 out]
                n3483 = local read "Com Port 3"() -> (w4749:refnum<visa-resource-name>)
                n3484 = call-poly "VISA Configure Serial Port"("VISA resource name"=w4749, "timeout (10sec)"=u32 1000, "termination char\n(0xA = '\\n' = LF)"=u8 10 ("termination char\n(0xA = '\\n' = LF)"), "Enable Termination\nChar (T)"=FALSE ("Enable Termination Char (T)"), "baud rate (9600)"="Humidity BaudRate", "data bits (8)"=u16 8 ("data bits"), "parity (0:none)"=w4756, "error in (no error)"=w4750, "stop bits (10: 1 bit)"=w4759, "flow control (0:none)"=w4760) -> ("VISA resource name out"=w4755:refnum<visa-resource-name>, "error out"=w4746:errorcluster)  [unwired: 4 in]
              }
            }
            n3485 = Compound Arithmetic op=AND(w4651, w4650, w4652) -> (w4649:bool)
            n3486 = case shown="True" w4649 {
              tunnel: w4648 -> [_ _]
              tunnel: w4657 -> [_ w4687]
              frame False {
              }
              frame True {
                w4685 = " " ("regular expression")
                n3487 = Match Pattern(string=w4687, regular expression=" ") -> (after substring=w4689:string)  [unwired: 1 in, 3 out]
                n3488 = Match Pattern(string=w4689, regular expression=w4685) -> (before substring=→"humid":string, after substring=w4686:string)  [unwired: 1 in, 2 out]
                n3489 = Match Pattern(string=w4686, regular expression=w4685) -> (before substring=→"temp_@Rh sensor":string)  [unwired: 1 in, 3 out]
              }
            }
            n3490 = local read "Quit"() -> (w4638:bool)
          }
          n3491 = VISA Close(VISA resource name=w4634, error in (no error)=w4635) -> (error out=w4631:errorcluster)
          n3492 = call <vilib>:"Clear Errors.vi"("error in (no error)"=w4631) -> ()  [unwired: 5 in, 2 out]
        }
        frame Enabled {
        }
      }
    }
    frame Enabled {
    }
  }
  n3493 = while {
    tunnel: [w4768] -> _
    i -> [w4768]
    stop <- w4763 stop-if-true
    # "Langauage selection"
    n3494 = property on="FF Calibration g" class="WFGraph (strict)"("Plot Area:Colors:FG Color"=u32 0) -> ()  [unwired: 2 in, 2 out]
    n3495 = Equal?(x="Lan flag", y=22.0) -> ()  [unwired: 1 out]
    n3496 = disable-structure shown="Disabled" {
      frame Disabled {
        n3497 = stacked-sequence {
          frame #0 {
            n3498 = case shown="\"Russian\"" "Language Selection" {
              tunnel: [0 1] -> w4770
              frame "English", Default {
              }
              frame "Russian" {
              }
            }
            n3499 = for {
              N: 130 -> [_]
              tunnel: "Table" -> [w4779]
              tunnel: w4770 -> [w4778]
              i -> [w4777]
              n3500 = Index Array(array=w4779, index (row)=w4777, index (col)=w4778) -> (element=w4776:string)
              n3501 = case shown="4" w4777 {
                tunnel: w4776 -> [w4780 w4781 _ w4782 w4783 w4784 w4785 w4786 w4787 w4788 w4789 w4790 w4791 w4792 w4793 w4794 w4795 w4796 w4797 w4798 w4799 w4800 w4801 w4802 w4803 w4804 w4805 w4806 w4807 _ _ w4808 w4809 w4810 w4811 w4812 w4813 w4822 w4829 w4836 w4843 w4847 w4850 w4853 w4855 w4857 w4858 w4859 w4860 w4861 w4862 w4863 w4864 w4865 w4866 w4867 w4868 w4869 w4870 w4871 w4872 w4873 w4874 w4875 w4876 w4877 w4878 w4879 w4880 w4881 w4882 w4883 w4884 w4885 w4886 w4887 w4888 w4889 w4890 w4891 w4892 w4893 w4894 w4895 w4896 w4897 w4898 w4899 w4900 w4901 w4902 w4903 w4904 w4905 w4906 w4907 w4908 w4909 w4910 w4911 w4912 w4913 w4914 w4915 w4916 _ w4917 w4918 w4919 w4920 w4921 w4922 w4923 w4924 w4925 w4926 w4927 w4928 w4929 _ w4930 w4931 w4932 w4933 w4934 w4935 _]
                frame 0 {
                  n3502 = local write "S"(w4780) -> ()
                }
                frame 1 {
                  n3503 = local write "S 2"(w4781) -> ()
                }
                frame 2 {
                }
                frame 3 {
                  n3504 = local write "S 4"(w4782) -> ()
                }
                frame 4 {
                  n3505 = property on="FILE" class="Str"("Caption.Text"=w4783) -> ()  [unwired: 2 in, 2 out]
                }
                frame 5 {
                  n3506 = property on="Fuel Discription :" class="Str"("Caption.Text"=w4784) -> ()  [unwired: 2 in, 2 out]
                }
                frame 6 {
                  n3507 = property on="Remarks :" class="Str"("Caption.Text"=w4785) -> ()  [unwired: 2 in, 2 out]
                }
                frame 7 {
                  n3508 = property on="Save & Continue" class="Bool (strict)"("Boolean Text.Text"=w4786) -> ()  [unwired: 2 in, 2 out]
                }
                frame 8 {
                }
                frame 9 {
                  n3509 = property on="Set Hz" class="DigNum (strict)"("Caption.Text"=w4788) -> ()  [unwired: 2 in, 2 out]
                }
                frame 10 {
                  "String 3" <- w4789
                }
                frame 11 {
                  n3510 = property on="NORMAL LOAD" class="DigNum (strict)"("Caption.Text"=w4790) -> ()  [unwired: 2 in, 2 out]
                }
                frame 12 {
                  "String 5" <- w4791
                }
                frame 13 {
                  n3511 = property on="Set Temp" class="DigNum (strict)"("Caption.Text"=w4792) -> ()  [unwired: 2 in, 2 out]
                }
                frame 14 {
                  n3512 = local write "S 15"(w4793) -> ()
                }
                frame 15 {
                  n3513 = property on="Set Rh" class="DigNum (strict)"("Caption.Text"=w4794) -> ()  [unwired: 2 in, 2 out]
                }
                frame 16 {
                  "String 13" <- w4795
                  "String 26" <- w4795
                }
                frame 17 {
                  n3514 = local write "S 18"(w4796) -> ()
                }
                frame 18 {
                  "String 17" <- w4797
                }
                frame 19 {
                  n3515 = property on="test time" class="DigNum (strict)"("Caption.Text"=w4798) -> ()  [unwired: 2 in, 2 out]
                }
                frame 20 {
                  "String 18" <- w4799
                  "String 22" <- w4799
                }
                frame 21 {
                  n3516 = property on="Elapsed time" class="DigNum (strict)"("Caption.Text"=w4800) -> ()  [unwired: 2 in, 2 out]
                }
                frame 22 {
                  n3517 = property on="Samplingtime 2" class="DigNum (strict)"("Caption.Text"=w4801) -> ()  [unwired: 2 in, 2 out]
                }
                frame 23 {
                  "String 21" <- w4802
                }
                frame 24 {
                  n3518 = property on="Countdown" class="DigNum (strict)"("Caption.Text"=w4803) -> ()  [unwired: 2 in, 2 out]
                }
                frame 25 {
                  n3519 = property on="Countdown 2" class="DigNum (strict)"("Caption.Text"=w4804) -> ()  [unwired: 2 in, 2 out]
                }
                frame 26 {
                  n3520 = property on="Engage" class="Bool (strict)"("Boolean Text.Text"=w4805) -> ()  [unwired: 2 in, 2 out]
                }
                frame 27 {
                  n3521 = property on="Boolean  4" class="Bool (strict)"("Boolean Text.Text"=w4806) -> ()  [unwired: 2 in, 2 out]
                }
                frame 28 {
                  n3522 = property on="Test \nStatus" class="Bool (strict)"("Boolean Text.Text"=w4807) -> ()  [unwired: 2 in, 2 out]
                }
                frame 29 {
                }
                frame 30 {
                }
                frame 31 {
                  n3523 = property on="FF Calibration g" class="WFGraph (strict)"("X Scale.Name Label.Text"=w4808) -> ()  [unwired: 2 in, 2 out]
                }
                frame 32 {
                  n3524 = property on="RSTCOF" class="Bool"("Boolean Text.Text"=w4809) -> ()  [unwired: 2 in, 2 out]
                  n3525 = property on="RST FF" class="Bool"("Boolean Text.Text"=w4809) -> ()  [unwired: 2 in, 2 out]
                  n3526 = property on="RST TEMP" class="Bool"("Boolean Text.Text"=w4809) -> ()  [unwired: 2 in, 2 out]
                  n3527 = property on="RSTV1 3" class="Bool"("Boolean Text.Text"=w4809) -> ()  [unwired: 2 in, 2 out]
                  n3528 = property on="rstv2" class="Bool"("Boolean Text.Text"=w4809) -> ()  [unwired: 2 in, 2 out]
                  n3529 = property on="RSTV1 2" class="Bool"("Boolean Text.Text"=w4809) -> ()  [unwired: 2 in, 2 out]
                  n3530 = property on="RST CP" class="Bool"("Boolean Text.Text"=w4809) -> ()  [unwired: 2 in, 2 out]
                }
                frame 33 {
                  "S 61" <- w4810
                }
                frame 34 {
                  "String 23" <- w4811
                }
                frame 35 {
                  n3531 = property on="Rh Before" class="DigNum (strict)"("Caption.Text"=w4812) -> ()  [unwired: 2 in, 2 out]
                }
                frame 36 {
                  n3532 = Match Pattern(string=w4813, regular expression=",") -> (before substring=→"bs":string, after substring=→"as":string)  [unwired: 1 in, 2 out]
                  n3533 = property on="Rh After" class="DigNum (strict)"("Caption.Text"=w4813) -> ()  [unwired: 2 in, 2 out]
                }
                frame 37 {
                  n3534 = Match Pattern(string=w4822, regular expression=",") -> (before substring=w4821:string, after substring=w4820:string)  [unwired: 1 in, 2 out]
                  "bs" <- w4821
                  "as" <- w4820
                  n3535 = Concatenate Strings(w4821, w4820) -> (w4817:string)
                  n3536 = property on="Humidity before test 2" class="DigNum (strict)"("Caption.Text"=w4817) -> ()  [unwired: 2 in, 2 out]
                  n3537 = property on="Humidity before test" class="DigNum (strict)"("Caption.Text"=w4817) -> ()  [unwired: 2 in, 2 out]
                  n3538 = Concatenate Strings(w4817, "=" ("string")) -> (w4818:string)
                  n3539 = local write "S 38"(w4818) -> ()
                }
                frame 38 {
                  n3540 = Match Pattern(string=w4829, regular expression=",") -> (before substring=w4828:string, after substring=w4827:string)  [unwired: 1 in, 2 out]
                  "bs" <- w4828
                  "as" <- w4827
                  n3541 = Concatenate Strings(w4828, w4827) -> (w4824:string)
                  n3542 = property on="Humidity after test 2" class="DigNum (strict)"("Caption.Text"=w4824) -> ()  [unwired: 2 in, 2 out]
                  n3543 = Concatenate Strings(w4824, "=" ("string")) -> (w4826:string)
                  n3544 = property on="Humidity after test" class="DigNum (strict)"("Caption.Text"=w4824) -> ()  [unwired: 2 in, 2 out]
                  n3545 = local write "S 39"(w4826) -> ()
                }
                frame 39 {
                  n3546 = Match Pattern(string=w4836, regular expression=",") -> (before substring=w4835:string, after substring=w4834:string)  [unwired: 1 in, 2 out]
                  "bs" <- w4835
                  "as" <- w4834
                  n3547 = Concatenate Strings(w4835, w4834) -> (w4831:string)
                  n3548 = property on="Temperature before test 2" class="DigNum (strict)"("Caption.Text"=w4831) -> ()  [unwired: 2 in, 2 out]
                  n3549 = property on="Temperature before test" class="DigNum (strict)"("Caption.Text"=w4831) -> ()  [unwired: 2 in, 2 out]
                  n3550 = Concatenate Strings(w4831, "=" ("string")) -> (→"String 34":string)
                }
                frame 40 {
                  n3551 = Match Pattern(string=w4843, regular expression=",") -> (before substring=w4842:string, after substring=w4841:string)  [unwired: 1 in, 2 out]
                  "bs" <- w4842
                  "as" <- w4841
                  n3552 = Concatenate Strings(w4842, w4841) -> (w4838:string)
                  n3553 = property on="Temperature after test 2" class="DigNum (strict)"("Caption.Text"=w4838) -> ()  [unwired: 2 in, 2 out]
                  n3554 = Concatenate Strings(w4838, "=" ("string")) -> (→"String 35":string)
                  n3555 = property on="Temperature after test" class="DigNum (strict)"("Caption.Text"=w4838) -> ()  [unwired: 2 in, 2 out]
                }
                frame 41 {
                  n3556 = property on="AVP" class="DigNum (strict)"("Caption.Text"=w4847) -> ()  [unwired: 2 in, 2 out]
                  n3557 = property on="AVP 2" class="DigNum (strict)"("Caption.Text"=w4847) -> ()  [unwired: 2 in, 2 out]
                  n3558 = Concatenate Strings(w4847, "=" ("string")) -> (→"String 36":string)
                }
                frame 42 {
                  n3559 = property on="MWSD" class="DigNum (strict)"("Caption.Text"=w4850) -> ()  [unwired: 2 in, 2 out]
                  n3560 = property on="MWSD 2" class="DigNum (strict)"("Caption.Text"=w4850) -> ()  [unwired: 2 in, 2 out]
                  n3561 = Concatenate Strings(w4850, "=" ("string")) -> (→"String 37":string)
                }
                frame 43 {
                  n3562 = property on="HCF 2" class="DigNum (strict)"("Caption.Text"=w4853) -> ()  [unwired: 2 in, 2 out]
                  n3563 = property on="HCF" class="DigNum (strict)"("Caption.Text"=w4853) -> ()  [unwired: 2 in, 2 out]
                  n3564 = Concatenate Strings(w4853, "=" ("string")) -> (→"String 38":string)
                }
                frame 44 {
                  n3565 = Concatenate Strings(w4855, "=" ("string")) -> (→"String 39":string)
                  n3566 = property on="WS1.4 2" class="DigNum (strict)"("Caption.Text"=w4855) -> ()  [unwired: 2 in, 2 out]
                  n3567 = property on="WS1.4" class="DigNum (strict)"("Caption.Text"=w4855) -> ()  [unwired: 2 in, 2 out]
                }
                frame 45 {
                  n3568 = property on="Save Results" class="Bool (strict)"("Boolean Text.Text"=w4857) -> ()  [unwired: 2 in, 2 out]
                }
                frame 46 {
                  n3569 = local write "S 47"(w4858) -> ()
                }
                frame 47 {
                  n3570 = local write "S 48"(w4859) -> ()
                }
                frame 48 {
                  n3571 = local write "S 49"(w4860) -> ()
                }
                frame 49 {
                  n3572 = local write "S 50"(w4861) -> ()
                }
                frame 50 {
                  n3573 = local write "S 51"(w4862) -> ()
                }
                frame 51 {
                  n3574 = local write "S 52"(w4863) -> ()
                }
                frame 52 {
                  n3575 = local write "S 53"(w4864) -> ()
                }
                frame 53 {
                  n3576 = local write "S 54"(w4865) -> ()
                }
                frame 54 {
                  n3577 = local write "S 55"(w4866) -> ()
                }
                frame 55 {
                  n3578 = local write "S 56"(w4867) -> ()
                }
                frame 56 {
                  n3579 = local write "S 57"(w4868) -> ()
                }
                frame 57 {
                  n3580 = local write "S 58"(w4869) -> ()
                }
                frame 58 {
                  n3581 = local write "S 59"(w4870) -> ()
                }
                frame 59 {
                  n3582 = local write "S 60"(w4871) -> ()
                }
                frame 60 {
                  n3583 = local write "S 62"(w4872) -> ()
                }
                frame 61 {
                  n3584 = local write "S 63"(w4873) -> ()
                }
                frame 62 {
                  n3585 = local write "S 64"(w4874) -> ()
                }
                frame 63 {
                  n3586 = local write "S 65"(w4875) -> ()
                }
                frame 64 {
                  n3587 = local write "S 66"(w4876) -> ()
                }
                frame 65 {
                  n3588 = local write "S 67"(w4877) -> ()
                }
                frame 66 {
                  n3589 = local write "S 68"(w4878) -> ()
                }
                frame 67 {
                  n3590 = local write "S 69"(w4879) -> ()
                }
                frame 68 {
                  n3591 = local write "S 70"(w4880) -> ()
                }
                frame 69 {
                  n3592 = local write "S 71"(w4881) -> ()
                }
                frame 70 {
                  n3593 = local write "S 72"(w4882) -> ()
                }
                frame 71 {
                  n3594 = local write "S 73"(w4883) -> ()
                }
                frame 72 {
                  n3595 = local write "S 74"(w4884) -> ()
                }
                frame 73 {
                  n3596 = local write "S 75"(w4885) -> ()
                }
                frame 74 {
                  n3597 = local write "S 76"(w4886) -> ()
                }
                frame 75 {
                  n3598 = local write "S 77"(w4887) -> ()
                }
                frame 76 {
                  n3599 = local write "S 78"(w4888) -> ()
                }
                frame 77 {
                  n3600 = local write "S 79"(w4889) -> ()
                }
                frame 79 {
                  n3601 = property on="Sample Temperature ( °C )" class="XYGraph (strict)"("Y Scale.Name Label.Text"=w4890) -> ()  [unwired: 2 in, 2 out]
                }
                frame 80 {
                  n3602 = local write "S 81"(w4891) -> ()
                  n3603 = property on="Humidity ( %RH )" class="XYGraph (strict)"("Y Scale.Name Label.Text"=w4891) -> ()  [unwired: 2 in, 2 out]
                }
                frame 78 {
                  n3604 = property on="Air Temperature  ( °C )" class="XYGraph (strict)"("X Scale.Name Label.Text"=w4892) -> ()  [unwired: 2 in, 2 out]
                  n3605 = property on="Humidity ( %RH )" class="XYGraph (strict)"("X Scale.Name Label.Text"=w4892) -> ()  [unwired: 2 in, 2 out]
                  n3606 = property on="Sample Temperature ( °C )" class="XYGraph (strict)"("X Scale.Name Label.Text"=w4892) -> ()  [unwired: 2 in, 2 out]
                  n3607 = property on="Coefficient Of Friction" class="XYGraph (strict)"("X Scale.Name Label.Text"=w4892) -> ()  [unwired: 2 in, 2 out]
                }
                frame 81 {
                  n3608 = property on="Air Temperature  ( °C )" class="XYGraph (strict)"("Y Scale.Name Label.Text"=w4893) -> ()  [unwired: 2 in, 2 out]
                }
                frame 82 {
                  n3609 = local write "S 84"(w4894) -> ()
                }
                frame 83 {
                  n3610 = local write "S 85"(w4895) -> ()
                }
                frame 84 {
                  n3611 = local write "S 86"(w4896) -> ()
                }
                frame 85 {
                  n3612 = local write "S 87"(w4897) -> ()
                }
                frame 86 {
                  n3613 = local write "S 88"(w4898) -> ()
                }
                frame 87 {
                  n3614 = property on="FF Calibration g" class="WFGraph (strict)"("Y Scale.Name Label.Text"=w4899) -> ()  [unwired: 2 in, 2 out]
                }
                frame 88 {
                  n3615 = local write "S 90"(w4900) -> ()
                }
                frame 89 {
                  n3616 = local write "S 91"(w4901) -> ()
                }
                frame 90 {
                  n3617 = local write "S 92"(w4902) -> ()
                }
                frame 91 {
                  n3618 = local write "S 93"(w4903) -> ()
                }
                frame 92 {
                  n3619 = local write "S 94"(w4904) -> ()
                }
                frame 93 {
                  n3620 = local write "S 95"(w4905) -> ()
                }
                frame 94 {
                  n3621 = local write "S 96"(w4906) -> ()
                }
                frame 95 {
                  n3622 = local write "S 97"(w4907) -> ()
                }
                frame 96 {
                  n3623 = local write "S 98"(w4908) -> ()
                }
                frame 97 {
                  n3624 = local write "S 99"(w4909) -> ()
                }
                frame 98 {
                  n3625 = local write "S 100"(w4910) -> ()
                }
                frame 99 {
                  n3626 = local write "S 101"(w4911) -> ()
                }
                frame 100 {
                  n3627 = local write "S 102"(w4912) -> ()
                }
                frame 101 {
                  n3628 = local write "S 103"(w4913) -> ()
                }
                frame 102 {
                  n3629 = local write "S 104"(w4914) -> ()
                }
                frame 103 {
                  n3630 = local write "S 105"(w4915) -> ()
                }
                frame 104 {
                  n3631 = local write "S 106"(w4916) -> ()
                }
                frame 105 {
                }
                frame 106 {
                  n3632 = property on="OK Button 17" class="Bool (strict)"("Boolean Text.Text"=w4917) -> ()  [unwired: 2 in, 2 out]
                }
                frame 107 {
                  n3633 = property on="OK Button 16" class="Bool (strict)"("Boolean Text.Text"=w4918) -> ()  [unwired: 2 in, 2 out]
                }
                frame 108 {
